vi "Comparaison_string.vi"(8 "Ligne en cours":string[][](array[string])=[["CMOD 1", "", "NA", "NA", "", "La valeur attendue est : C88SZEN42_SW_V1.0.177995"], ["CMOD 2", "", "NA", "NA", "", "La valeur attendue est : C88SZEN42_SW_V1.0.177995"], ["PDU", "", "NA", "NA", "", "La valeur attendue est : PWBX_SW_APP_V0009.04.00B "], ["BMS", "", "NA", "NA", "", "La valeur attendue est : UEGB_SW_APP_V160036.0011_01"]], 9 "offset lecture valeur":string, 10 "valeur attendue":string, 11 "Valeur lue":string) -> (1 "PASS / FAIL":bool, 3 "output array":string[][](array[string]))   [LabVIEW 2017]
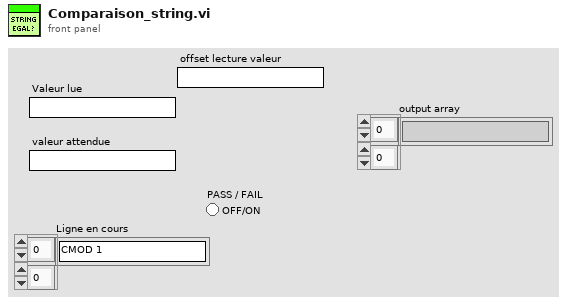
[diagram p1: front panel]
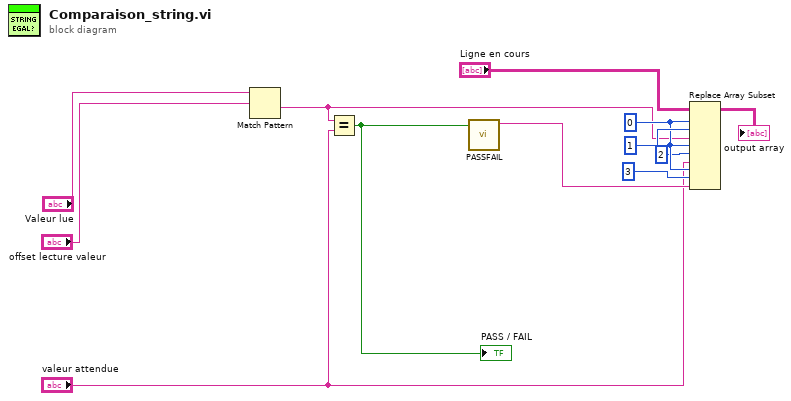
[diagram p0: block diagram]
diagram:
  w5 = 0 ("index (row)")
  n1 = Match Pattern(string="Valeur lue", regular expression="offset lecture valeur") -> (after substring=w1:string)  [unwired: 1 in, 3 out]
  n2 = Equal?(x=w1, y="valeur attendue") -> (x = y?=w12:bool)
  "PASS / FAIL" <- w12
  n3 = call "PASSFAIL.vi"("E"=w12) -> ("S"=w6:string)  [unwired: 10 in]
  n4 = Replace Array Subset(array="Ligne en cours", new element #1=w1, index (row) #1=w5, index (col) #1=1 ("disabled index (col)"), new element #2="valeur attendue", index (row) #2=w5, index (col) #2=2 ("disabled index (col)"), new element #3=w6, index (row) #3=w5, index (col) #3=3 ("disabled index (col)")) -> (→"output array":string[][])
